vi "WS1021 VCmin Header.vi"(8 "Error In":errorcluster) -> (0 "Error Out":errorcluster, 3 "VCmin CS Header":string[](array[string]))   [LabVIEW 2017]
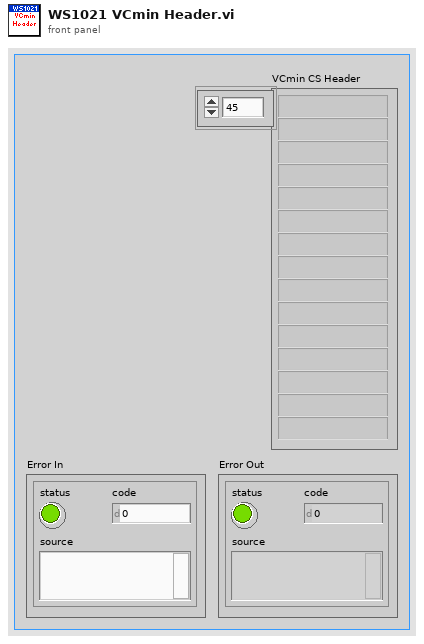
[diagram p1: front panel]
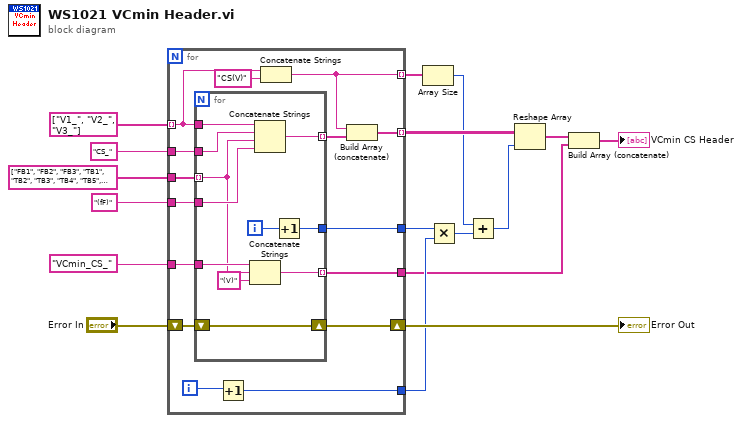
[diagram p0: block diagram]
diagram:
  n1 = for {
    tunnel: string[] ["FB1", "FB2", "FB3", "TB1", "TB2", "TB3", "TB4", "TB5", "TB6", "TB7", "TB8", "TB9", "TB10", "TB11"] -> [w32]
    tunnel: "CS_" ("string") -> [w31]
    tunnel: "(fF)" ("string") -> [w30]
    tunnel: [w21] -> w10 mode=indexing
    shift-right: [w28] -> w13
    shift-left: "Error In" -> [w29]
    tunnel: string[] ["V1_", "V2_", "V3_"] -> [w20] mode=indexing
    tunnel: [w27] -> w7
    tunnel: [w25] -> w8
    tunnel: "VCmin_CS_" -> [w24]
    tunnel: [w23] -> w5
    tunnel: [w18] -> w3 mode=indexing
    i -> [w26]
    n2 = for {
      tunnel: w32 -> [w35] mode=indexing
      tunnel: [w43] -> w22 mode=indexing
      tunnel: w31 -> [w42]
      tunnel: w30 -> [w41]
      shift-right: [w40] -> w28
      shift-left: w29 -> [w40]
      tunnel: w20 -> [w39]
      tunnel: [w37] -> w27
      tunnel: w24 -> [w36]
      tunnel: [w34] -> w23 mode=indexing
      i -> [w38]
      n3 = Concatenate Strings(w36, w35, "(V)" ("string")) -> (w34:string)
      n4 = Concatenate Strings(w39, w42, w35, w41) -> (w43:string)
      n5 = Increment(x=w38) -> (x+1=w37:i32)
    }
    n6 = Increment(x=w26) -> (x+1=w25:i32)
    n7 = Concatenate Strings(w20, "CS(V)" ("string")) -> (w18:string)
    n8 = Build Array (concatenate)(w18, w22) -> (w21:string[])
  }
  "Error Out" <- w13
  n9 = Array Size(array=w3) -> (size(s)=w2:i32)
  n10 = Multiply(x=w7, y=w8) -> (x*y=w4:i32)
  n11 = Add(x=w2, y=w4) -> (x+y=w1:i32)
  n12 = Reshape Array(w10, w1) -> (w9:string[])
  n13 = Build Array (concatenate)(w9, w5) -> (→"VCmin CS Header":string[])
